vi "Create Plugins.vi"(8 "error in (no error)":errorcluster, 9 "async plugins tag":string, 10 "inline plugins tag":string, 11 "Application Data In":T1) -> (0 "error out":errorcluster, 2 "avg bandwidth":dbl, 3 "Application Data out":T1)   [LabVIEW 2017, in "DSF Core.lvlib"]
uses:
  DSF Core.lvlib
  Main VI/Application Data.ctl
  LabVIEW-Memory/Source/Classes/Pointer/Pointer.lvclass
  Classes/Framework/Framework.lvclass
  Buffer Reader/Buffer Data.ctl
  Classes/Buffer/Buffer.lvclass
  C:/Git/DSF/LabVIEW-Memory/Source/Classes/Pointer/Pointer.lvclass
  Classes/Transfer Group Status/Status.lvclass
  Typedefs/DSF Data Type.ctl
  Typedefs/DSF Engine Channel Configuration.ctl
  Typedefs/DSF Settings Info.ctl
  Typedefs/DSF Byte Order.ctl
  Typedefs/DSF Engine Framework Configuration.ctl
  Typedefs/DSF Engine Plugin Configuration.ctl
  Typedefs/DSF Timing Info.ctl
  Typedefs/DSF Engine Plugin Thread Configuration.ctl
  Typedefs/DSF Engine Transfer Group Configuration.ctl
  Typedefs/DSF Direction.ctl
  Typedefs/DSF Engine Transfer Configuration.ctl
  Typedefs/DSF Timeout Behavior.ctl
  Classes/Framework/Framework.lvclass/Framework.ctl
  Classes/Framework Status/Framework Status.lvclass/Framework Status.ctl
  Classes/Plugin/Plugin.lvclass/Plugin.ctl
  Classes/Timing/Timing.lvclass/Timing.ctl
  Classes/Transfer Group/Transfer Group.lvclass/Transfer Group.ctl
  Classes/Buffers/Buffers.lvclass/Buffers.ctl
  Classes/Transfer/Transfer.lvclass/Transfer.ctl
  Classes/Plugin/Get Name.vi
  Create New Tree Item.vi
  Add Transfer Group with Children.vi
  Classes/Plugin/Get Inline Tx Transfer Groups.vi
  Classes/Plugin/Get Timing.vi
  Classes/Timing/Get Decimation.vi
  Classes/Plugin/Get Buffers.vi
  Classes/Buffers/Get String Buffer.vi
  Classes/Transfer Group/Sort Groups by ID.vi
  Classes/Plugin/Get Inline Rx Transfer Groups.vi
  Classes/Plugin/Get Async Tx Transfer Groups.vi
  Classes/Plugin/Get Async Rx Transfer Groups.vi
  Classes/Transfer Group/Get Name.vi
  Add Transfer with Children.vi
  Classes/Transfer Group/Get Transfers.vi
  Classes/Transfer Group/Get Inline.vi
  Classes/Transfer Group/Get Timing.vi
  Classes/Transfer Group/Get Buffers.vi
  Buffer Reader/Average Cycle Bandwidth.vi
  Classes/Transfer/Get Name.vi
  Classes/Transfer/Get Buffers.vi
  Add Buffers with Children.vi
  Classes/Buffer/Get Buffer Size.vi
  Classes/Buffers/Get Inline Buffer.vi
  Classes/Buffers/Get Async Buffer.vi
  Add Buffer Channels.vi
  Sizeof.vi
  Add Item to Tree.vi
  LabVIEW-Memory/Source/Classes/Pointer/Get Size.vi
  Classes/Buffer/Subset Buffer.vi
  Classes/Framework Status/Framework Status.lvclass
  Classes/Plugin/Plugin.lvclass
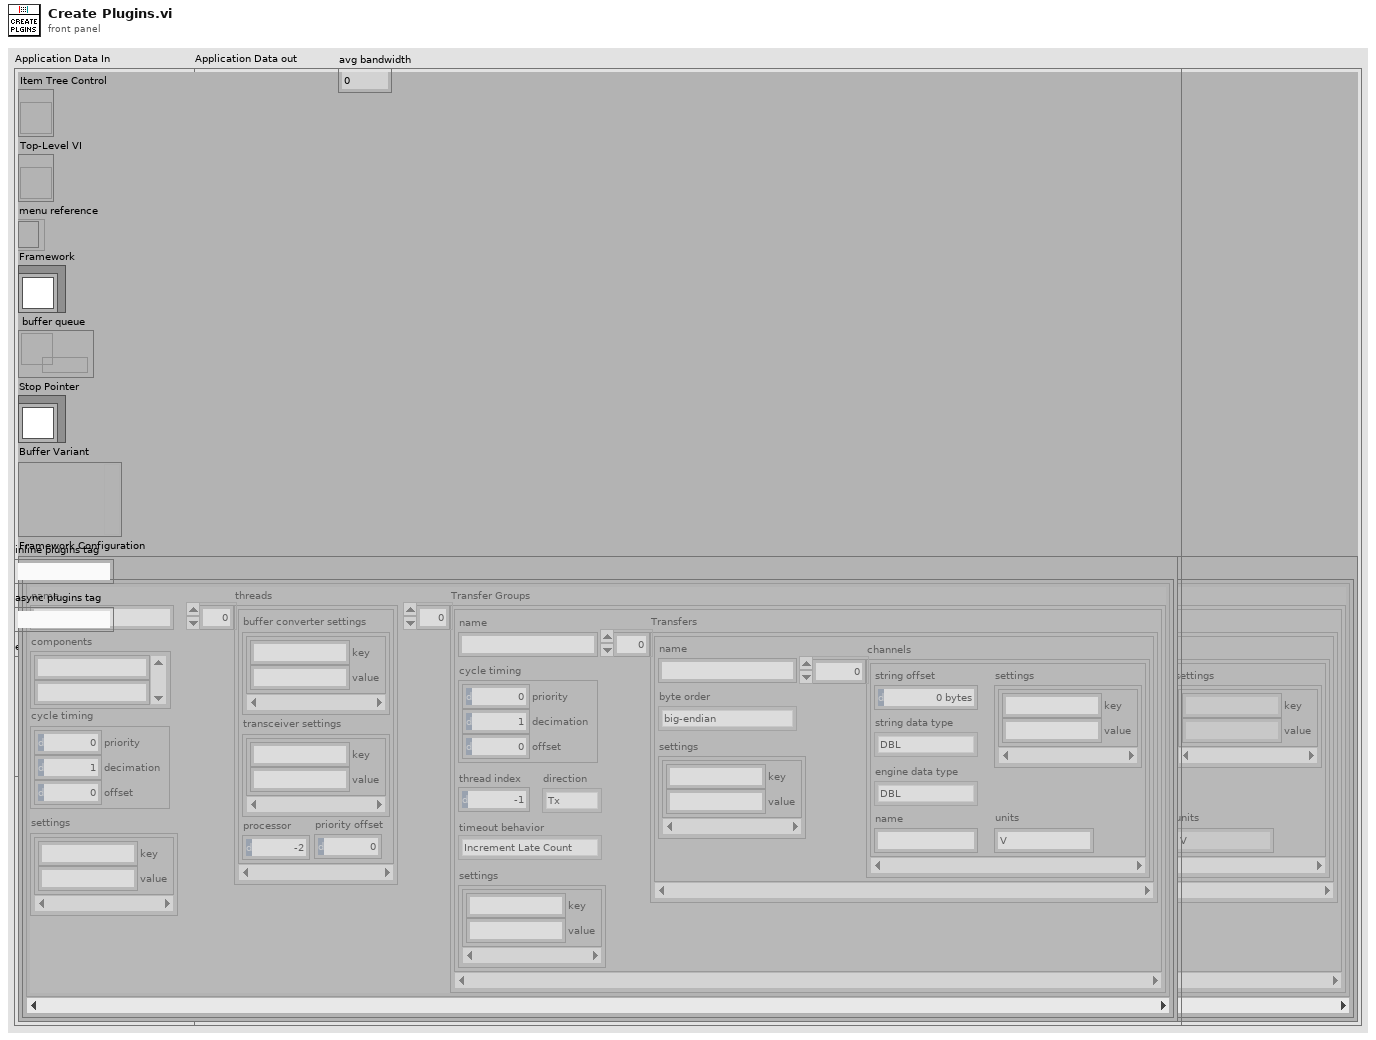
[diagram p1: front panel]
types:
  T1 = typedef "DSF Core.lvlib/Application Data.ctl" = cluster{"Item Tree Control":refnum<vi>, "Top-Level VI":refnum<vi>, "menu reference":refnum<k9>, "Framework":refnum<class "Framework.lvclass">, "buffer queue":refnum<queue>, "Stop Pointer":refnum<class "Pointer.lvclass">, "Buffer Variant":variant, "Framework Configuration":T2}
  T2 = typedef "DSF Core.lvlib/DSF Engine Framework Configuration.ctl" = cluster{"Plugins":T3[]}
  T3 = typedef "DSF Core.lvlib/DSF Engine Plugin Configuration.ctl" = cluster{"name":string, "components":string[], "cycle timing":T4, "threads":T5[], "Transfer Groups":T7[], "settings":T6}
  T4 = typedef "DSF Core.lvlib/DSF Timing Info.ctl" = cluster{"priority":u64, "decimation":u64, "offset":u64}
  T5 = typedef "DSF Core.lvlib/DSF Engine Plugin Thread Configuration.ctl" = cluster{"buffer converter settings":T6, "transceiver settings":T6, "processor":i32, "priority offset":i16}
  T6 = typedef "DSF Core.lvlib/DSF Settings Info.ctl" = cluster{"key":string, "value":string}[]
  T7 = typedef "DSF Core.lvlib/DSF Engine Transfer Group Configuration.ctl" = cluster{"name":string, "direction":T8, "cycle timing":T4, "thread index":i32, "settings":T6, "Transfers":T9[], "timeout behavior":T13}
  T8 = typedef "DSF Core.lvlib/DSF Direction.ctl" = enum8{"Tx", "Rx"}
  T9 = typedef "DSF Core.lvlib/DSF Engine Transfer Configuration.ctl" = cluster{"name":string, "byte order":T10, "settings":T6, "channels":T11[]}
  T10 = typedef "DSF Core.lvlib/DSF Byte Order.ctl" = enum8{"big-endian", "little-endian"}
  T11 = typedef "DSF Core.lvlib/DSF Engine Channel Configuration.ctl" = cluster{"string offset":u64, "string data type":T12, "engine data type":T12, "name":string, "settings":T6, "units":string}
  T12 = typedef "DSF Core.lvlib/DSF Data Type.ctl" = enum8{"Bool", "SGL", "DBL", "I8", "I16", "I32", "I64", "U8", "U16", "U32", "U64"}
  T13 = typedef "DSF Core.lvlib/DSF Timeout Behavior.ctl" = enum8{"Increment Late Count", "Throw Error"}
  T14 = typedef "DSF Core.lvlib/Buffer Data.ctl" = cluster{"Buffer":refnum<class "Buffer.lvclass">, "Status":refnum<class "Status.lvclass">, "decimation":u64, "avg bandwidth":dbl, "data type":T12, "units":string, "channels":T11[], "channel":bool, "engine (T) / string (F)":bool, "byte order":T10}
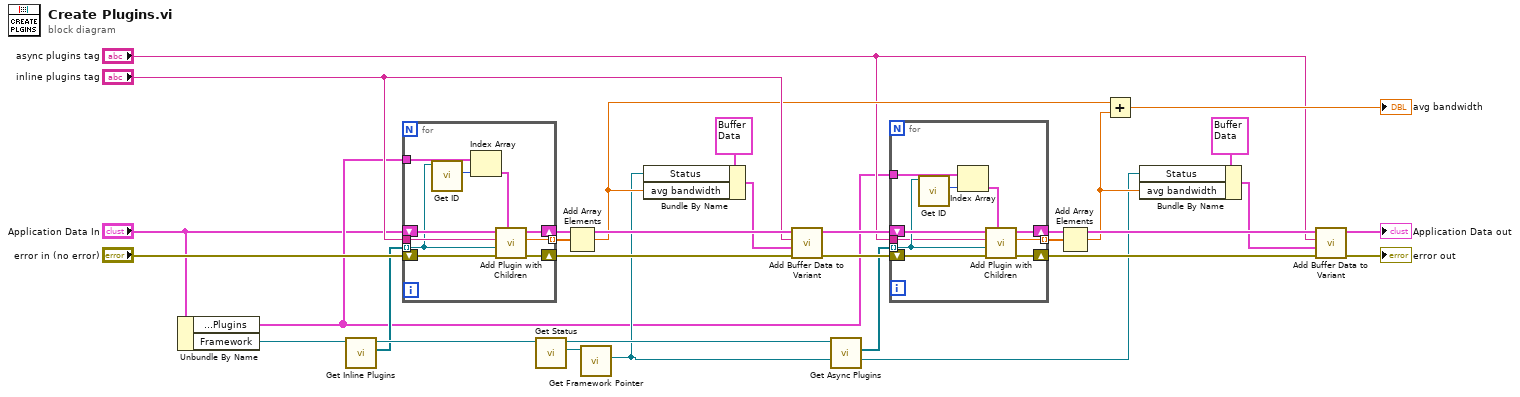
[diagram p0: block diagram]
diagram:
  n1 = Unbundle By Name("Application Data In") -> ("Framework Configuration.Plugins"=w2:T3[], "Framework"=w7:refnum<class "Framework.lvclass">)
  n2 = call "Get Inline Plugins.vi"("Framework in"=w7) -> ("Inline Plugins"=w5:refnum<class "Plugin.lvclass">[], "Framework out"=w6:refnum<class "Framework.lvclass">)  [unwired: 9 in]
  n3 = for {
    shift-right: [w36] -> w24
    shift-left: "error in (no error)" -> [w38]
    tunnel: w5 -> [w32] mode=indexing
    tunnel: "inline plugins tag" -> [w33]
    shift-right: [w37] -> w25
    shift-left: "Application Data In" -> [w39]
    tunnel: [w35] -> w28 mode=indexing
    tunnel: w2 -> [w34]
    n4 = call "Get ID.vi"("Plugin in"=w32) -> ("id"=w31:i32)  [unwired: 9 in, 1 out]
    n5 = Index Array(array=w34, index=w31) -> (element=w30:T3)
    n6 = call "Add Plugin with Children.vi"("Plugin configuration"=w30, "error in (no error)"=w38, "Plugin"=w32, "parent tag"=w33, "Application Data In"=w39) -> ("error out"=w36:errorcluster, "average bandwidth"=w35:dbl, "Application Data Out"=w37:T1)  [unwired: 4 in]
  }
  n7 = call "Get Status.vi"("Framework in"=w6) -> ("Status"=w9:refnum<class "Framework Status.lvclass">, "Framework out"=w4:refnum<class "Framework.lvclass">)  [unwired: 9 in]
  n8 = Add Array Elements(numeric array=w28) -> (sum=w14:dbl)
  n9 = call "Get Framework Pointer.vi"("Framework Status in"=w9) -> ("framework pointer"=w3:refnum<class "Status.lvclass">)  [unwired: 9 in, 1 out]
  n10 = Bundle By Name(cluster=T14 {"Buffer"=refnum, "Status"=refnum, "decimation"=0, "avg bandwidth"=0.0, "data type"=enum."Bool", "units"="", "channels"=[], "channel"=FALSE, "engine (T) / string (F)"=FALSE, "byte order"=enum."little-endian"} ("Buffer data"), "Status"=w3, "avg bandwidth"=w14) -> (w15:T14)
  n11 = call "Add Buffer Data to Variant.vi"("error in (no error)"=w24, "Buffer data"=w15, "tag"="inline plugins tag", "Application Data In in"=w25) -> ("error out"=w22:errorcluster, "Application Data In out"=w23:T1)  [unwired: 6 in]
  n12 = call "Get Async Plugins.vi"("Framework in"=w4) -> ("Async Plugins"=w13:refnum<class "Plugin.lvclass">[])  [unwired: 9 in, 1 out]
  n13 = for {
    shift-right: [w46] -> w19
    shift-left: w22 -> [w48]
    shift-right: [w47] -> w21
    shift-left: w23 -> [w49]
    tunnel: "async plugins tag" -> [w40]
    tunnel: w13 -> [w41] mode=indexing
    tunnel: [w45] -> w27 mode=indexing
    tunnel: w2 -> [w43]
    n14 = call "Get ID.vi"("Plugin in"=w41) -> ("id"=w44:i32)  [unwired: 9 in, 1 out]
    n15 = Index Array(array=w43, index=w44) -> (element=w42:T3)
    n16 = call "Add Plugin with Children.vi"("Plugin configuration"=w42, "error in (no error)"=w48, "Plugin"=w41, "parent tag"=w40, "Application Data In"=w49) -> ("error out"=w46:errorcluster, "average bandwidth"=w45:dbl, "Application Data Out"=w47:T1)  [unwired: 4 in]
  }
  n17 = Add Array Elements(numeric array=w27) -> (sum=w11:dbl)
  n18 = Add(x=w14, y=w11) -> (x+y=→"avg bandwidth":dbl)
  n19 = Bundle By Name(cluster=T14 {"Buffer"=refnum, "Status"=refnum, "decimation"=0, "avg bandwidth"=0.0, "data type"=enum."Bool", "units"="", "channels"=[], "channel"=FALSE, "engine (T) / string (F)"=FALSE, "byte order"=enum."little-endian"} ("Buffer data"), "Status"=w3, "avg bandwidth"=w11) -> (w10:T14)
  n20 = call "Add Buffer Data to Variant.vi"("error in (no error)"=w19, "Buffer data"=w10, "tag"="async plugins tag", "Application Data In in"=w21) -> ("error out"=→"error out":errorcluster, "Application Data In out"=→"Application Data out":T1)  [unwired: 6 in]
